vi "System Close.vi"(8 "error in (no error)":errorcluster) -> (0 "error out":errorcluster)   [LabVIEW 2013]
uses:
  Image Acquisition/Host Image Acquisition Module Enum.ctl
  Message Passing/Main MsgQ.lvlib
  Common/Utility/Utility Lib.lvlib
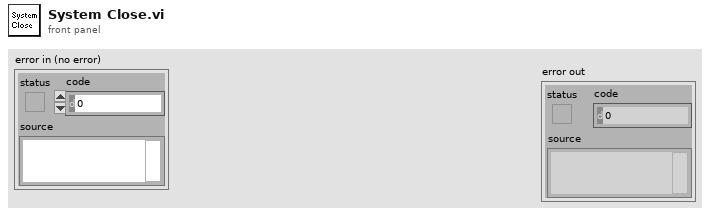
[diagram p1: front panel]
types:
  T1 = typedef "Host Image Acquisition Module Enum.ctl" = enum16{"Open FPGA", "Initialize DMA FIFO", "Load Sim Images", "Initialize Acquisition", "Update Sector Parameters", "Start Acquisition", "Aquire Image", "Read Averages", "Cancel Acquisition", "Close FPGA"}
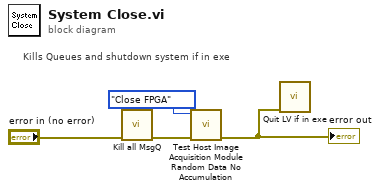
[diagram p0: block diagram]
diagram:
  # "Kills Queues and shutdown system if in exe"
  n1 = call "Kill all MsgQ.vi"("error in (no error)"="error in (no error)") -> ("error out"=w2:errorcluster)  [unwired: 10 out]
  n2 = call "Test Host Image Acquisition Module Random Data No Accumulation.vi"("error in"=w2, "Operation"=Host_Image_Acquisition_Module_Enum."Close FPGA") -> ("error out"=w1:errorcluster)  [unwired: 6 in, 3 out]
  "error out" <- w1
  n3 = call "Quit LV if in exe.vi"("error in (no error)"=w1) -> ()  [unwired: 11 out]
